vi "Polar to Cartesian.vi"(8 "Scale":dbl=0.01, 9 "Resulotion":i32, 11 "LIDAR Data":cluster{"Magnitude":dbl[], "Direction":dbl[]}) -> (0 "XY":cluster{dbl[], dbl[]}, 3 "LIDAR Data scaled rad":cluster{"Magnitude":dbl[], "Direction":dbl[]})   [LabVIEW 2011]
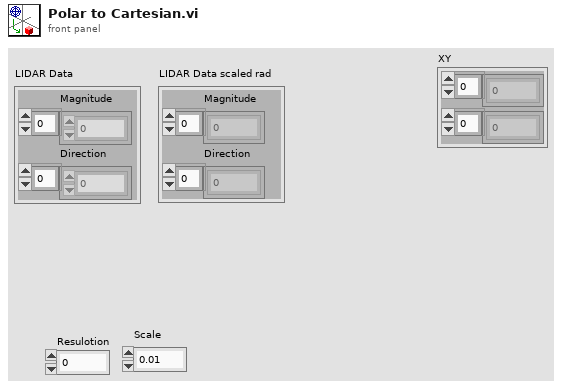
[diagram p1: front panel]
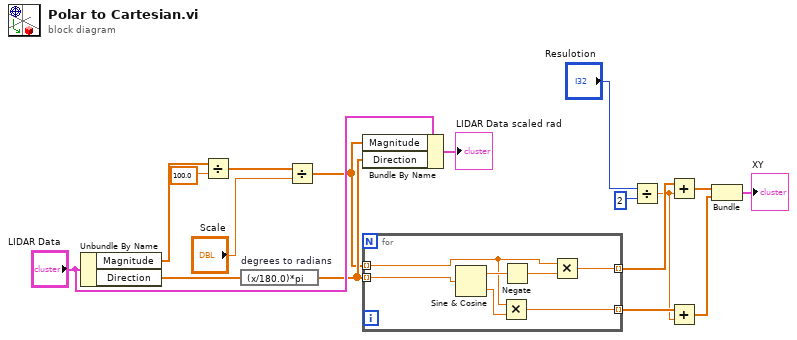
[diagram p0: block diagram]
diagram:
  n1 = Unbundle By Name("LIDAR Data") -> ("Magnitude"=w6:dbl[], "Direction"=w17:dbl[])
  n2 = Divide(x=w6, y=100.0 ("Scale")) -> (x/y=w4:dbl[])
  n3 = expression code="(x/180.0)*pi" "degrees to radians"(w17) -> (w8:dbl[])
  n4 = Divide(x=w4, y="Scale") -> (x/y=w2:dbl[])
  n5 = Bundle By Name(cluster="LIDAR Data", "Magnitude"=w2, "Direction"=w8) -> (→"LIDAR Data scaled rad":cluster{"Magnitude":dbl[], "Direction":dbl[]})
  n6 = for {
    tunnel: w2 -> [w19] mode=indexing
    tunnel: w8 -> [w20] mode=indexing
    tunnel: [w22] -> w16 mode=indexing
    tunnel: [w18] -> w14 mode=indexing
    n7 = Sine & Cosine(0:w20) -> (1:w24:dbl, 2:w23:dbl)
    n8 = Multiply(x=w19, y=w23) -> (x*y=w18:dbl)
    n9 = Negate(x=w24) -> (-x=w21:dbl)
    n10 = Multiply(x=w19, y=w21) -> (x*y=w22:dbl)
  }
  n11 = Divide(x="Resulotion", y=2) -> (x/y=w11:dbl)
  n12 = Add(x=w16, y=w11) -> (x+y=w15:dbl[])
  n13 = Add(x=w14, y=w11) -> (x+y=w13:dbl[])
  n14 = Bundle(w15, w13) -> (→"XY":cluster{dbl[], dbl[]})  [unwired: 1 out]
